vi "Read SHV Setpoint.vi"(8 "error in (no error)":errorcluster, 11 "Stepper in":refnum<class "Stepper.lvclass">) -> (0 "error out":errorcluster, 2 "data out":dbl, 3 "Stepper out":refnum<class "Stepper.lvclass">)   [LabVIEW 2015, in "Stepper.lvclass"]
uses:
  Stepper.lvclass
  Stepper.lvclass/Stepper.ctl
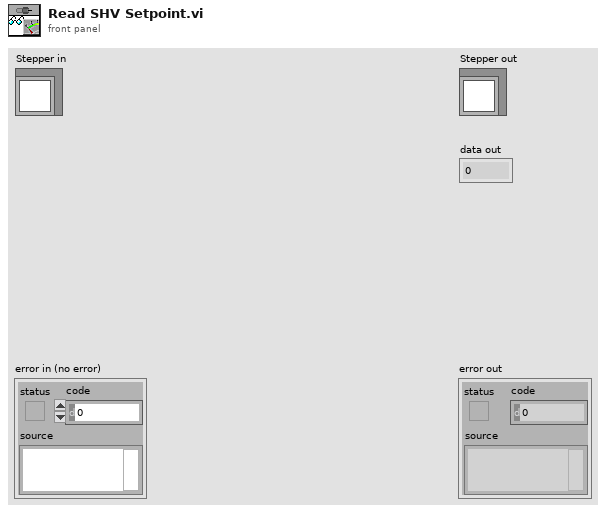
[diagram p1: front panel]
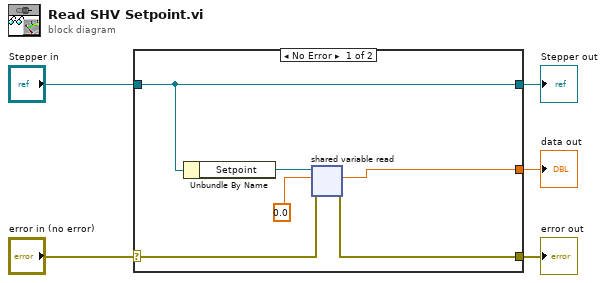
[diagram p0: block diagram]
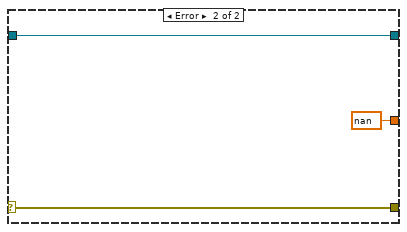
[diagram p2: hidden frame]
diagram:
  n1 = case shown="No Error" "error in (no error)" {
    selector: "error in (no error)" -> [w9 w13]
    tunnel: [w8 w13] -> w4
    tunnel: [w11 w14] -> w2
    tunnel: "Stepper in" -> [w11 w14]
    tunnel: [w6 nan] -> w1
    frame No Error {
      n2 = Unbundle By Name(w11) -> ("Setpoint"=w10:refnum<k21>)
      n3 = shared-variable-read(w10, w9, 0.0) -> (w8:errorcluster, w6:dbl)  [unwired: 2 out]
    }
    frame Error {
    }
  }
  "error out" <- w4
  "Stepper out" <- w2
  "data out" <- w1
